vi "Pre-Build Action.vi"(6 "Top Level/Always Included VIs":path[](array[path]), 7 "Main Destination Path":path, 9 "Target Name":string, 10 "Build Specification Name":string, 11 "Project Path":path) -> (0 "error out":errorcluster)   [LabVIEW 2017]
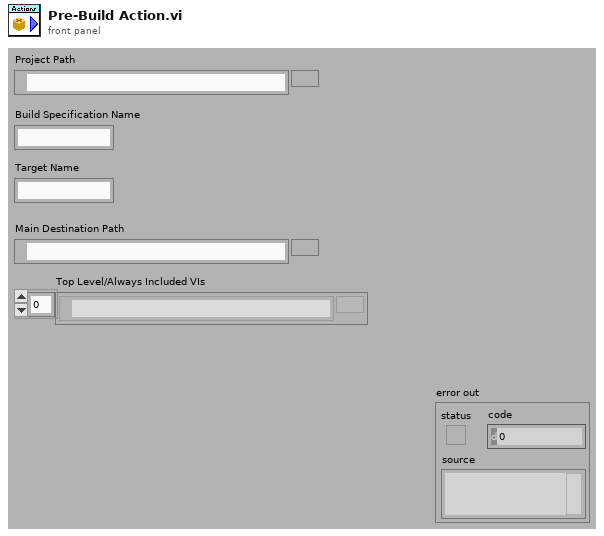
[diagram p1: front panel]
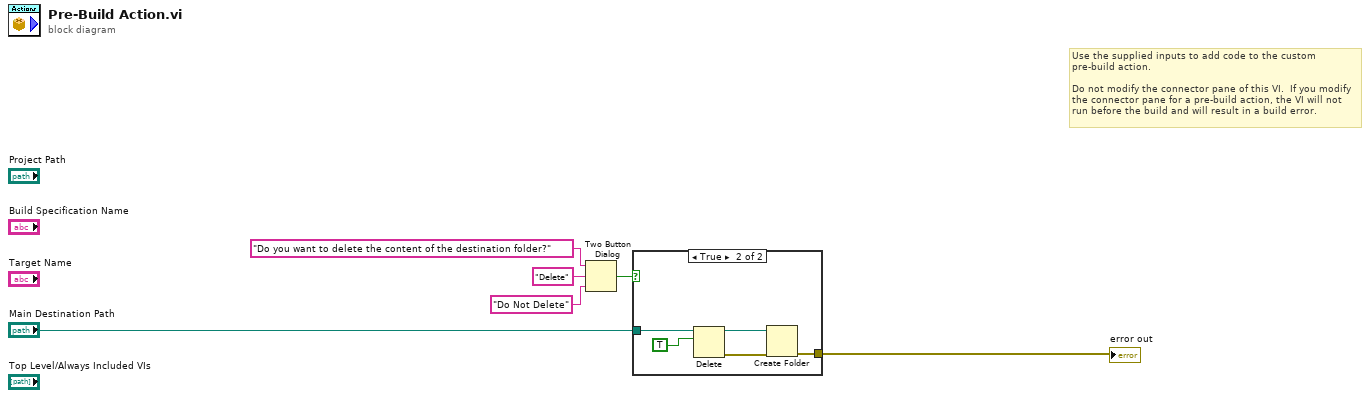
[diagram p0: block diagram]
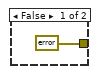
[diagram p2: hidden frame]
diagram:
  # "Use the supplied inputs to add code to the custom pre-build action.\n\nDo not modify the connector pane of this VI.  If you modify the connector pane for a pre-build action, the VI will not run before the build and will result in a build error."
  n1 = Two Button Dialog(message="Do you want to delete the content of the destination folder?", 1:"Do Not Delete" ("F button name (\"Cancel\")"), 2:"Delete" ("T button name (\"OK\")")) -> (T button?=w3:bool)
  n2 = case shown="True" w3 {
    tunnel: [errorcluster {"status"=FALSE, "code"=0, "source"=""} ("error in (no error)") w9] -> w2
    tunnel: "Main Destination Path" -> [_ w12]
    frame False {
    }
    frame True {
      n3 = Delete(path (use dialog)=w12, entire hierarchy (F)=TRUE) -> (deleted path=w8:path, error out=w10:errorcluster)  [unwired: 3 in, 1 out]
      n4 = Create Folder(path (use dialog)=w8, error in=w10) -> (error out=w9:errorcluster)  [unwired: 1 in, 2 out]
    }
  }
  "error out" <- w2
